vi "normalizeXMLname.vi"(10 "Input Attribute Name":string) -> (2 "Compliant Attribute Name":string)   [LabVIEW 2020, in "Caraya.lvlib" / "MsgSerializer.XML.lvclass"]
uses:
  MsgSerializer.XML.lvclass
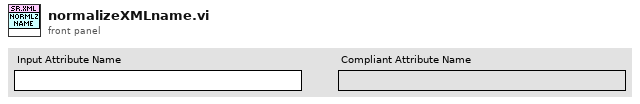
[diagram p1: front panel]
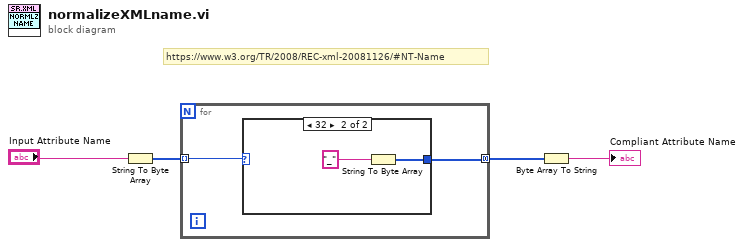
[diagram p0: block diagram]
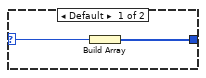
[diagram p2: hidden frame]
diagram:
  # "https://www.w3.org/TR/2008/REC-xml-20081126/#NT-Name"
  n1 = String To Byte Array(string="Input Attribute Name") -> (unsigned byte array=w3:u8[])
  n2 = for {
    tunnel: w3 -> [w6] mode=indexing
    tunnel: [w5] -> w1 mode=concatenating
    n3 = case shown="32" w6 {
      selector: w6 -> [w8 _]
      tunnel: [w7 w10] -> w5
      frame Default {
        n4 = Build Array(w8) -> (w7:u8[])
      }
      frame 32 {
        n5 = String To Byte Array(string="_" ("Input String")) -> (unsigned byte array=w10:u8[])
      }
    }
  }
  n6 = Byte Array To String(unsigned byte array=w1) -> (string=→"Compliant Attribute Name":string)
